vi "Clear.vi"(8 "error in (no error)":errorcluster, 11 "Gantry 2":refnum<k24>) -> (0 "error out":errorcluster, 3 "Gantry 3":refnum<k24>)   [LabVIEW 2020, in "Motion.lvclass"]
uses:
  Motion.lvclass
  C:/Program Files (x86)/Aerotech/A3200/LabVIEW/2010/Bin/Aerotech.A3200.dll
  Program Files (x86)/Aerotech/A3200/LabVIEW/2010/Bin/Aerotech.A3200.dll
  A3200/A3200.lvclass
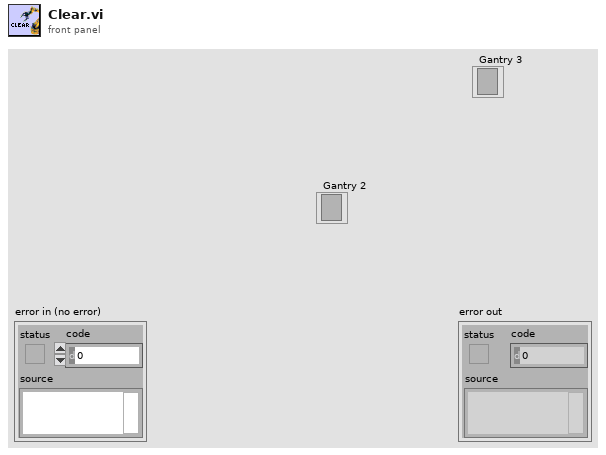
[diagram p1: front panel]
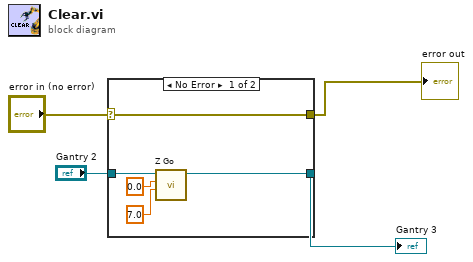
[diagram p0: block diagram]
diagram:
  n1 = case shown="No Error" "error in (no error)" {
    selector: "error in (no error)" -> [w9 w11]
    tunnel: [w9 w11] -> w3
    tunnel: [w5 w10] -> w1
    tunnel: "Gantry 2" -> [w8 w10]
    frame No Error {
      n2 = call "Z Go.vi"("Speed"=7.0, "Position"=0.0, "Gantry 2"=w8) -> ("Gantry 3"=w5:refnum<k24>)  [unwired: 7 in, 1 out]
    }
    frame Error {
    }
  }
  "error out" <- w3
  "Gantry 3" <- w1
